vi "NI.AO.vi"(5 "测试日志信息":refnum<queue>, 6 "Freq":dbl=1000.0 min=1.0, 7 "amplitude":dbl=1.0 caption="幅值" format="%0.2p", 8 "error in":errorcluster caption="Error In", 9 "CMD":enum16{"OPEN AO", "CLOSE AO"}(ring), 10 "AO Channel":enum16{"AO0", "AO1"}(ring), 11 "DAQmx Device":tag="Dev1") -> (0 "error out":errorcluster caption="错误输出", 1 "Fs":dbl, 2 "SamplesPerChanl":u32 caption="每通道写入采样数", 4 "波形图表":waveform(dbl)(graph))   [LabVIEW 2012, in "Lib_UEL.ATE.lvlib" / "Lib_PCI6221.lvlib"]
uses:
  Lib_PCI6221.lvlib
  <vilib>/Utility/error.llb/DialogType.ctl
  <vilib>/DAQmx/write.llb/DAQmx Write (Analog Wfm 1Chan NSamp).vi
  <vilib>/DAQmx/create/channels.llb/DAQmx Create Channel (AO-Voltage-Basic).vi
  <vilib>/DAQmx/configure/timing.llb/DAQmx Timing (Sample Clock).vi
  <vilib>/DAQmx/miscellaneous.llb/DAQmx Fill In Error Info.vi
  <vilib>/measure/NI_MABase.lvlib
  <resource>/objmgr/daqmx.rc
panel:
  # "V01 - Initial Version. ~LI.Guang 2011-05-13 \n V02 - 2012/1/11, 增加日志功能, 使用队列."
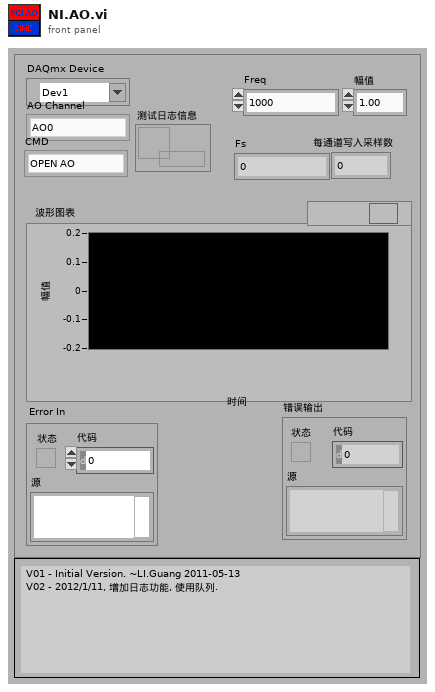
[diagram p1: front panel]
types:
  T1 = enum16{"Sine Wave", "Triangle Wave", "Square Wave", "Sawtooth Wave"}
  T2 = typedef "DialogType.ctl" = u16
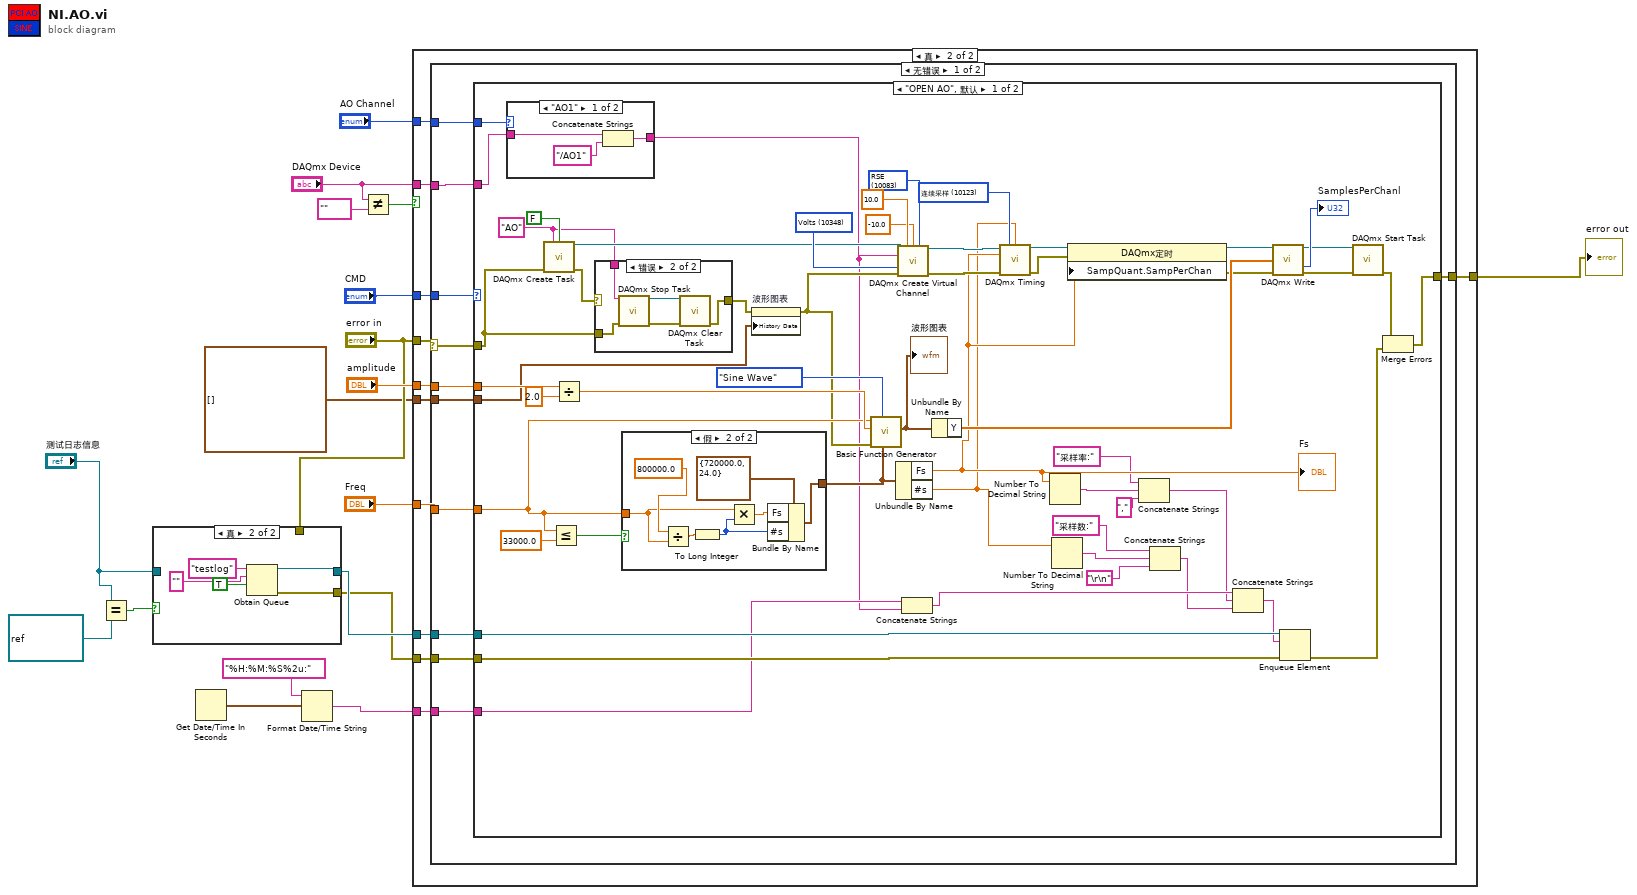
[diagram p0: block diagram]
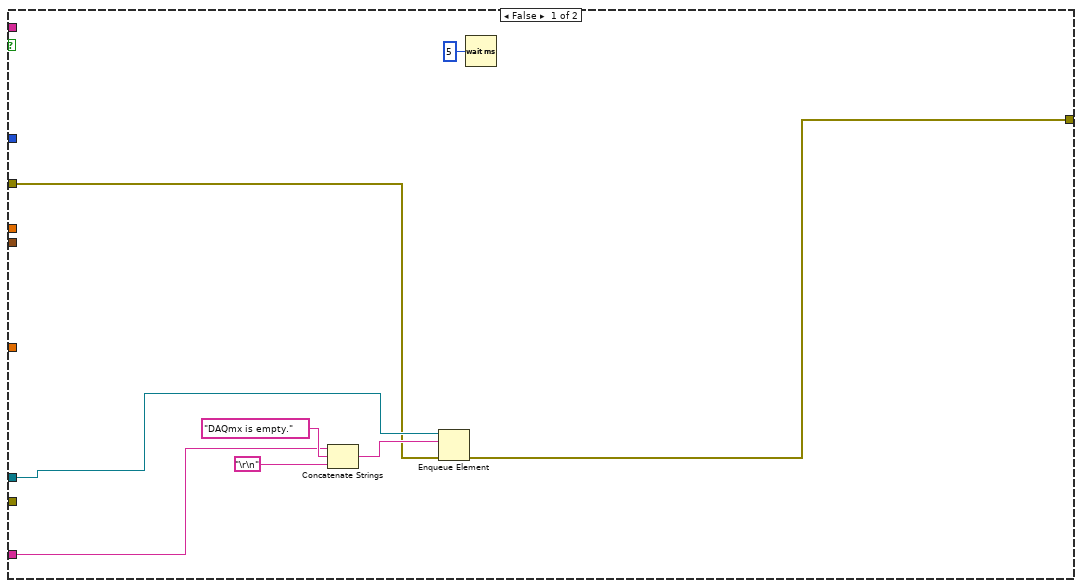
[diagram p3: hidden frame]
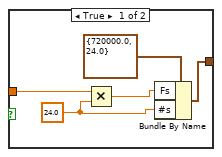
[diagram p5: hidden frame]
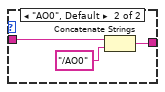
[diagram p6: hidden frame]
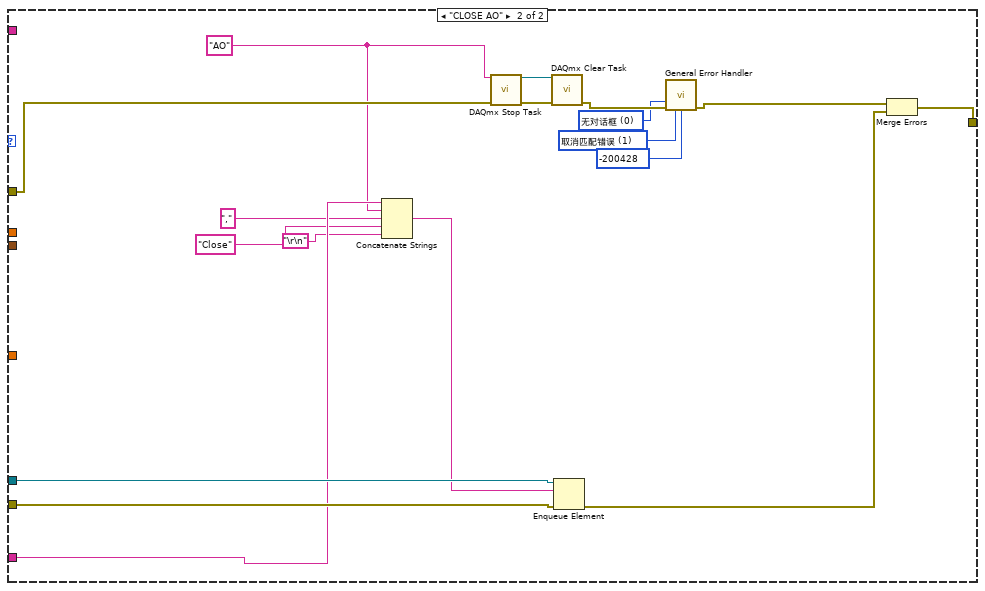
[diagram p7: hidden frame]
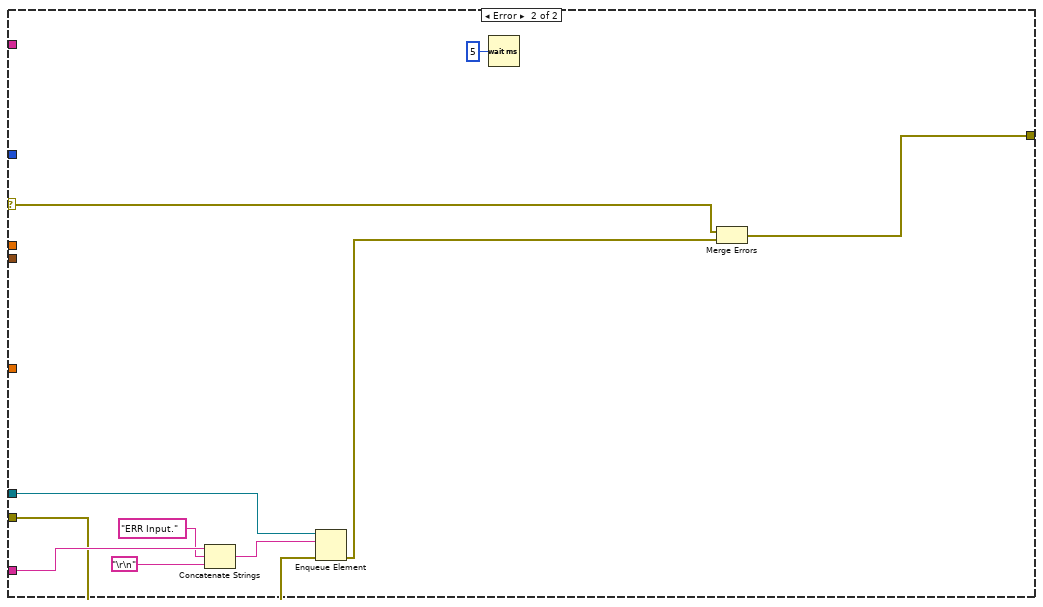
[diagram p8: hidden frame]
diagram:
  n1 = Equal?(x="测试日志信息", y=refnum<queue> refnum) -> (x = y?=w6:bool)
  n2 = case shown="真" w6 {
    tunnel: "测试日志信息" -> [w20 _]
    tunnel: [w20 w25] -> w4
    tunnel: [w19 w24] -> w2
    tunnel: "error in" -> [w19 _]
    frame False {
    }
    frame True {
      n3 = Obtain Queue(name (unnamed)="testlog" ("名称（未命名）"), element data type="" ("名称（未命名）"), create if not found? (T)=TRUE ("如未找到是否创建？(T)")) -> (queue out=w25:refnum<queue>, error out=w24:errorcluster)  [unwired: 2 in, 1 out]
    }
  }
  n4 = Get Date/Time In Seconds() -> (seconds since 1Jan1904=w9:timestamp)
  n5 = Format Date/Time String(time format string (%c)="%H:%M:%S%2u:" ("时间格式化字符串(%c)"), seconds (now)=w9) -> (date/time string=w8:string)  [unwired: 1 in]
  n6 = Not Equal?(x="DAQmx Device", y=tag "") -> (x != y?=w11:bool)
  n7 = case shown="真" w11 {
    tunnel: "error in" -> [w28 w44]
    tunnel: "AO Channel" -> [_ w43]
    tunnel: "Freq" -> [_ w42]
    tunnel: "amplitude" -> [_ w41]
    tunnel: "CMD" -> [_ w40]
    tunnel: [w27 w39] -> w14
    tunnel: "DAQmx Device" -> [_ w38]
    tunnel: w4 -> [w30 w37]
    tunnel: w8 -> [w29 w36]
    tunnel: w2 -> [_ w35]
    tunnel: waveform(dbl)[] [] ("历史数据") -> [_ w34]
    frame False {
      n8 = Concatenate Strings(w29, "DAQmx is empty." ("字符串"), "\r\n") -> (w32:string)
      n9 = Enqueue Element(queue=w30, element=w32, error in (no error)=w28) -> (error out=w27:errorcluster)  [unwired: 1 in, 2 out]
      n10 = Wait (ms)(milliseconds to wait=u32 5 ("等待时间（毫秒）")) -> ()  [unwired: 1 out]
    }
    frame True {
      n11 = case shown="无错误" w44 {
        selector: w44 -> [w48 w159]
        tunnel: w38 -> [w54 _]
        tunnel: w43 -> [w55 _]
        tunnel: w42 -> [w52 _]
        tunnel: w41 -> [w53 _]
        tunnel: [w51 w157] -> w39
        tunnel: w40 -> [w50 _]
        tunnel: w37 -> [w49 w160]
        tunnel: w36 -> [w47 w156]
        tunnel: w35 -> [w46 w151]
        tunnel: w34 -> [w45 _]
        frame No Error {
          n12 = case shown="\"OPEN AO\", 默认" w50 {
            tunnel: w48 -> [w56 w148]
            tunnel: w55 -> [w96 _]
            tunnel: w54 -> [w95 _]
            tunnel: w53 -> [w85 _]
            tunnel: w52 -> [w82 _]
            tunnel: [w61 w138] -> w51
            tunnel: w49 -> [w79 w147]
            tunnel: w46 -> [w78 w146]
            tunnel: w47 -> [w69 w145]
            tunnel: w45 -> [w60 _]
            frame "OPEN AO", Default {
              w89 = 10123 items=["有限采样"=10178, "连续采样"=10123, "硬件定时单点"=12522] ("sample mode")
              w102 = 10083 items=["默认"=-1, "RSE"=10083, "差分"=10106, "伪差分"=12529] ("output terminal configuration")
              w106 = 10348 items=["Volts"=10348, "来自自定义换算"=10065] ("units")
              w57 = "AO" ("new task name")
              n13 = case shown="\"AO1\"" w96 {
                tunnel: w95 -> [w128 w131]
                tunnel: [w127 w130] -> w68
                frame "AO1" {
                  n14 = Concatenate Strings(w128, "/AO1" ("new task name")) -> (w127:string)
                }
                frame "AO0", Default {
                  n15 = Concatenate Strings(w131, "/AO0" ("new task name")) -> (w130:string)
                }
              }
              n16 = call <vilib>:"DAQmx Create Task.vi"("new task name"=w57, "auto cleanup"=FALSE, "error in"=w56) -> ("task out"=w86:refnum<k21>, "error out"=w59:errorcluster)  [unwired: 11 in]
              n17 = Less Or Equal?(x=w82, y=33000.0) -> (x <= y?=w93:bool)
              n18 = Divide(x=w85, y=2.0) -> (x/y=w83:dbl)
              n19 = case shown="错误" w59 {
                selector: w59 -> [w109 _]
                tunnel: [w109 w110] -> w58
                tunnel: w57 -> [_ w112]
                tunnel: w56 -> [_ w111]
                frame No Error {
                }
                frame Error {
                  n20 = call <vilib>:"DAQmx Stop Task.vi"("task/channels in"=w112, "error in"=w111) -> ("task out"=w114:refnum<k21>, "error out"=w113:errorcluster)  [unwired: 12 in]
                  n21 = call <vilib>:"DAQmx Clear Task.vi"("task in"=w114, "error in"=w113) -> ("error out"=w110:errorcluster)  [unwired: 13 in]
                }
              }
              n22 = case shown="假" w93 {
                tunnel: [w118 w125] -> w97
                tunnel: w82 -> [w116 w122]
                frame True {
                  w117 = 24.0 ("Fs")
                  n23 = Multiply(x=w116, y=w117) -> (x*y=w115:dbl)
                  n24 = Bundle By Name(cluster=cluster{"Fs":dbl, "#s":dbl} {"Fs"=720000.0, "#s"=24.0} ("sampling info"), "Fs"=w115, "#s"=w117) -> (w118:cluster{"Fs":dbl, "#s":dbl})
                }
                frame False {
                  n25 = Divide(x=800000.0 ("Fs"), y=w122) -> (x/y=w121:dbl)
                  n26 = To Long Integer(number=w121) -> (32bit integer=w120:i32)
                  n27 = Multiply(x=w122, y=w120) -> (x*y=w124:dbl)
                  n28 = Bundle By Name(cluster=cluster{"Fs":dbl, "#s":dbl} {"Fs"=720000.0, "#s"=24.0} ("sampling info"), "Fs"=w124, "#s"=w120) -> (w125:cluster{"Fs":dbl, "#s":dbl})
                }
              }
              n29 = property on="波形图表" class="WFChart (严格)"(error in=w58, "History Data"=w60) -> (error out=w81:errorcluster)  [unwired: 1 in, 1 out]
              n30 = call <vilib>:"Basic Function Generator.vi"("sampling info"=w97, "signal type"=T1."Sine Wave", "error in (no error)"=w81, "amplitude"=w83, "frequency"=w82) -> ("signal out"=w99:waveform(dbl))  [unwired: 4 in, 2 out]
              "波形图表" <- w99
              n31 = Unbundle By Name(w97) -> ("Fs"=w77:dbl, "#s"=w74:dbl)
              "Fs" <- w77
              n32 = call-poly <vilib>:"DAQmx Create Virtual Channel.vi"("task in"=w86, "maximum value"=10.0 ("frequency"), "minimum value"=-10.0 ("amplitude"), "output terminal configuration"=w102, "physical channels"=w68, "units"=w106, "error in"=w81) -> ("task out"=w88:refnum<k21>, "error out"=w92:errorcluster)  [unwired: 7 in]
              n33 = Concatenate Strings(w69, w68) -> (w67:string)
              n34 = Unbundle By Name(w99) -> ("Y"=w100:dbl[])
              n35 = call-poly <vilib>:"DAQmx Timing.vi"("task/channels in"=w88, "sample mode"=w89, "samples per channel"=w74, "rate"=w77, "error in"=w92) -> ("task out"=w87:refnum<k21>, "error out"=w91:errorcluster)  [unwired: 9 in]
              n36 = Number To Decimal String(number=w77) -> (decimal integer string=w75:string)  [unwired: 1 in]
              n37 = Number To Decimal String(number=w74) -> (decimal integer string=w71:string)  [unwired: 1 in]
              n38 = property class="DAQmx定时"(reference=w87, error in=w91, "SampQuant.SampPerChan"=w77) -> (reference out=w98:refnum<k21>, error out=w90:errorcluster)
              n39 = Concatenate Strings("采样率:" ("时间格式化字符串(%c)"), w75, "," ("时间格式化字符串(%c)")) -> (w66:string)
              n40 = Concatenate Strings("采样数:" ("时间格式化字符串(%c)"), w71, "\r\n") -> (w65:string)
              n41 = Concatenate Strings(w67, w66, w65) -> (w64:string)
              n42 = call-poly <vilib>:"DAQmx Write.vi"("task/channels in"=w98, "data"=w100, "error in"=w90) -> ("task out"=w101:refnum<k21>, "number of samples written per channel"=→"SamplesPerChanl":u32, "error out"=w103:errorcluster)  [unwired: 10 in]
              n43 = Enqueue Element(queue=w79, element=w64, error in (no error)=w78) -> (error out=w63:errorcluster)  [unwired: 1 in, 2 out]
              n44 = call <vilib>:"DAQmx Start Task.vi"("task/channels in"=w101, "error in"=w103) -> ("error out"=w62:errorcluster)  [unwired: 12 in, 1 out]
              n45 = Merge Errors(w62, w63) -> (w61:errorcluster)
            }
            frame "CLOSE AO" {
              w133 = T2 0 items=["无对话框", "确定信息", "继续或停止信息", "确定信息＋警告", "继续/停止+警告"] ("type of dialog (OK msg:1)")
              w135 = 1 items=["无异常", "取消匹配错误", "设置匹配错误"] ("[exception action] (none:0)")
              w144 = "AO" ("new task name")
              n46 = Concatenate Strings(w145, w144, "," ("new task name"), "Close" ("new task name"), "\r\n") -> (w140:string)
              n47 = call <vilib>:"DAQmx Stop Task.vi"("task/channels in"=w144, "error in"=w148) -> ("task out"=w150:refnum<k21>, "error out"=w149:errorcluster)  [unwired: 12 in]
              n48 = call <vilib>:"DAQmx Clear Task.vi"("task in"=w150, "error in"=w149) -> ("error out"=w137:errorcluster)  [unwired: 13 in]
              n49 = Enqueue Element(queue=w147, element=w140, error in (no error)=w146) -> (error out=w139:errorcluster)  [unwired: 1 in, 2 out]
              n50 = call <vilib>:"General Error Handler.vi"("type of dialog (OK msg:1)"=w133, "error in (no error)"=w137, "[exception action] (none:0)"=w135, "[exception code]"=-200428 ("error code (no error:0)")) -> ("error out"=w134:errorcluster)  [unwired: 7 in, 4 out]
              n51 = Merge Errors(w134, w139) -> (w138:errorcluster)
            }
          }
        }
        frame Error {
          n52 = Concatenate Strings(w156, "ERR Input." ("字符串"), "\r\n") -> (w154:string)
          n53 = Enqueue Element(queue=w160, element=w154, error in (no error)=w151) -> (error out=w158:errorcluster)  [unwired: 1 in, 2 out]
          n54 = Wait (ms)(milliseconds to wait=u32 5 ("等待时间（毫秒）")) -> ()  [unwired: 1 out]
          n55 = Merge Errors(w159, w158) -> (w157:errorcluster)
        }
      }
    }
  }
  "error out" <- w14
